vi "GetEquipment.vi"(8 "error in (no error)":errorcluster, 11 "reference in":refnum<class "EquipmentVisitor.lvclass">) -> (0 "error out":errorcluster, 2 "Equipment":refnum<class "Equipment.lvclass">, 3 "reference out":refnum<class "EquipmentVisitor.lvclass">)   [LabVIEW 2020, in "EquipmentVisitor.lvclass"]
uses:
  EquipmentVisitor.lvclass
  Equipment_class/Equipment.lvclass
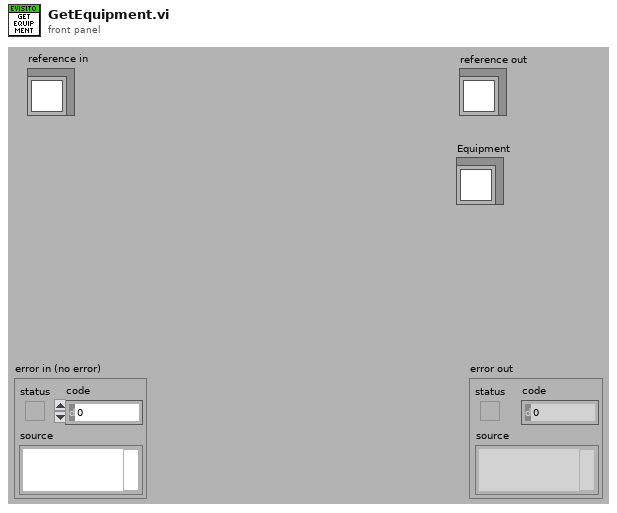
[diagram p1: front panel]
types:
  T1 = typedef "EquipmentVisitor.lvclass/ObjectAttributes.ctl" = cluster{"Equipment":refnum<class "Equipment.lvclass">}
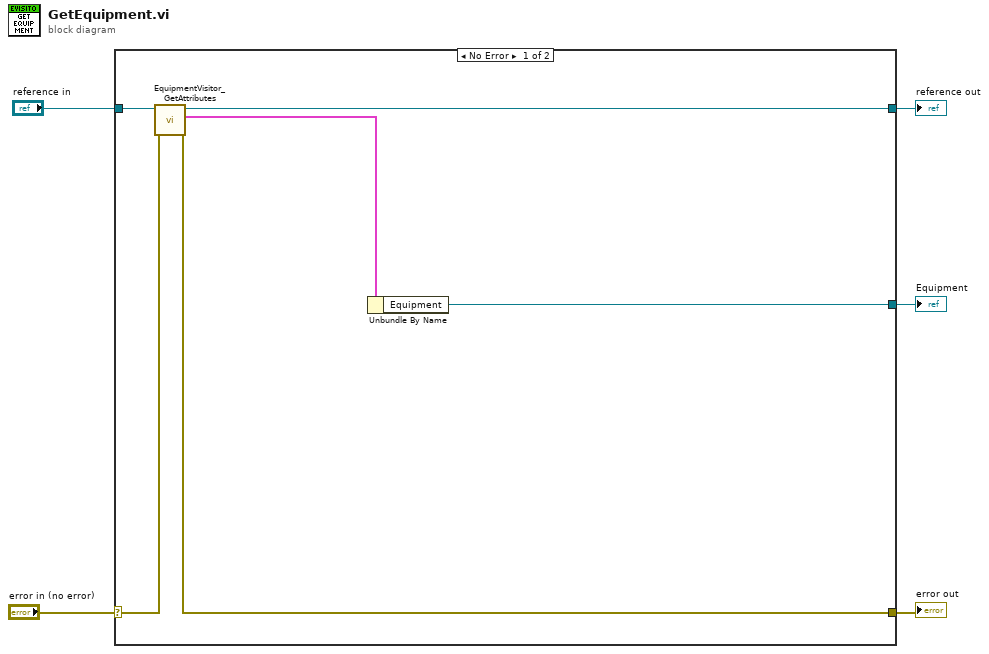
[diagram p0: block diagram]
diagram:
  n1 = case shown="No Error" "error in (no error)" {
    selector: "error in (no error)" -> [w11 w13]
    tunnel: [w9 w13] -> w4
    tunnel: [w7 w12] -> w2
    tunnel: "reference in" -> [w8 w12]
    tunnel: [w6 _] -> w1
    frame No Error {
      n2 = call "EquipmentVisitor_GetAttributes.vi"("error in (no error)"=w11, "reference in"=w8) -> ("error out"=w9:errorcluster, "Data"=w10:T1, "reference out"=w7:refnum<class "EquipmentVisitor.lvclass">)  [unwired: 6 in, 1 out]
      n3 = Unbundle By Name(w10) -> ("Equipment"=w6:refnum<class "Equipment.lvclass">)
    }
    frame Error {
    }
  }
  "error out" <- w4
  "reference out" <- w2
  "Equipment" <- w1
